vi "ITM10_get.vi"(7 "command":string="PR", 8 "error in":errorcluster, 11 "VISA_ref_in":refnum<visa-resource-name>="COM3") -> (0 "error out":errorcluster={"status"=TRUE, "code"=1, "source"="Scan From String (arg 1) in mks946_sub_get.vi"}, 3 "VISA_ref_out":refnum<visa-resource-name>="COM3", 4 "status":bool, 5 "response":string)   [LabVIEW 2019]
panel:
  out "bytes":u32
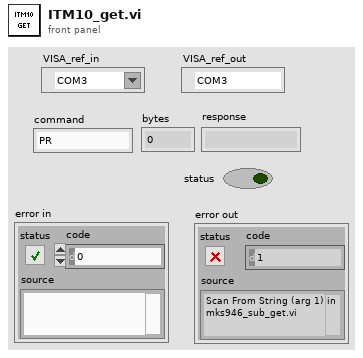
[diagram p1: front panel]
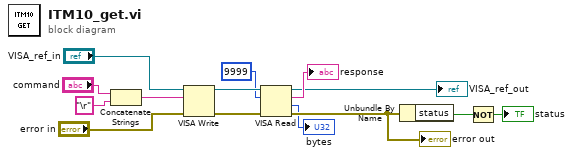
[diagram p0: block diagram]
diagram:
  n1 = Concatenate Strings("command", "\r" ("string")) -> (w4:string)
  n2 = VISA Write(VISA resource name="VISA_ref_in", write buffer=w4, error in (no error)="error in") -> (VISA resource name out=w6:refnum<visa-resource-name>, error out=w5:errorcluster)  [unwired: 1 out]
  n3 = VISA Read(VISA resource name=w6, byte count=u32 9999, error in (no error)=w5) -> (VISA resource name out=→"VISA_ref_out":refnum<visa-resource-name>, read buffer=→"response":string, return count=→"bytes":u32, error out=w11:errorcluster)
  "error out" <- w11
  n4 = Unbundle By Name(w11) -> ("status"=w12:bool)
  n5 = Not(x=w12) -> (.not. x?=→"status":bool)
